vi "Get Control References.vi"(8 "error in (no error)":errorcluster, 9 "Controls to Exclude":refnum<vi>[](array[refnum]), 11 "VI Refnum":refnum<vi>) -> (0 "error out":errorcluster, 2 "Controls":T1)   [LabVIEW 2015, in "AutoRegistration.lvlib" / "AutoRegistration.lvclass"]
uses:
  AutoRegistration.lvclass
  Registration References.ctl
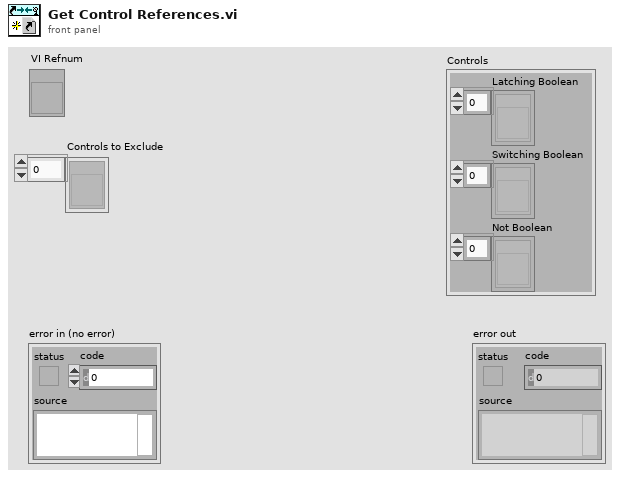
[diagram p1: front panel]
types:
  T1 = typedef "AutoRegistration.lvlib/AutoRegistration.lvclass/Registration References.ctl" = cluster{"Latching Boolean":refnum<vi>[], "Switching Boolean":refnum<vi>[], "Not Boolean":refnum<vi>[]}
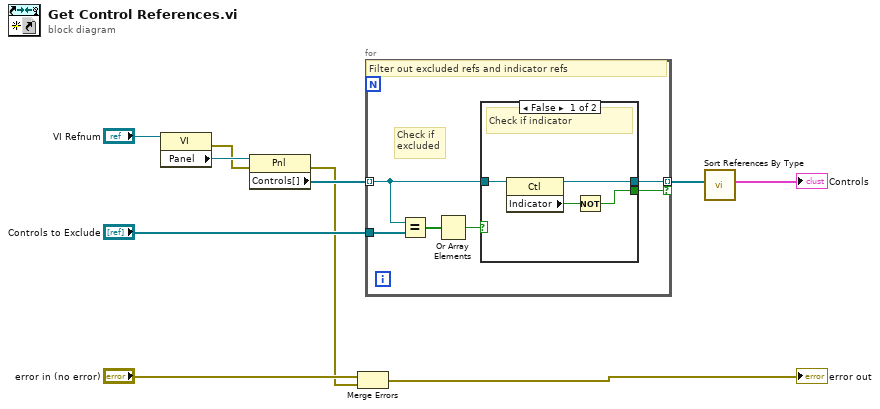
[diagram p0: block diagram]
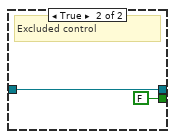
[diagram p2: hidden frame]
diagram:
  n1 = property class="VI"(reference="VI Refnum") -> (error out=w7:errorcluster, "Panel"=w8:refnum<vi>)  [unwired: 1 in, 1 out]
  n2 = property class="Pnl"(reference=w8, error in=w7) -> (error out=w1:errorcluster, "Controls[]"=w6:refnum<vi>[])  [unwired: 1 out]
  n3 = Merge Errors("error in (no error)", w1) -> (→"error out":errorcluster)
  n4 = for {
    tunnel: w6 -> [w12] mode=indexing
    tunnel: "Controls to Exclude" -> [w16]
    tunnel: [w11] -> w3 mode=indexing if=w13
    # "Check if\nexcluded"
    # "Filter out excluded refs and indicator refs"
    n5 = Equal?(x=w12, y=w16) -> (x = y?=w15:bool[])
    n6 = Or Array Elements(Boolean array=w15) -> (logical OR=w14:bool)
    n7 = case shown="False" w14 {
      tunnel: [w18 FALSE] -> w13
      tunnel: w12 -> [w20 w21]
      tunnel: [w17 w21] -> w11
      frame False {
        # "Check if indicator"
        n8 = property class="Ctl"(reference=w20) -> (reference out=w17:refnum<vi>, "Indicator"=w19:bool)  [unwired: 1 in, 1 out]
        n9 = Not(x=w19) -> (.not. x?=w18:bool)
      }
      frame True {
        # "Excluded control"
      }
    }
  }
  n10 = call "Sort References By Type.vi"("Controls to Register"=w3) -> ("Controls"=→"Controls":T1)  [unwired: 10 in]
